vi "get_base_frequency.vi"(8 "error in (no error)":errorcluster, 11 "DL090211FPGAWrapper in":refnum<class "FPGAWrapperDL090211Galvo_grabber.lvclass">) -> (0 "error out":errorcluster, 2 "base frequency":dbl[unit]=40000000.0, 3 "DL090211FPGAWrapper out":refnum<class "FPGAWrapperDL090211Galvo_grabber.lvclass">)   [LabVIEW 2010, in "FPGAWrapperDL090211Galvo_grabber.lvclass"]
uses:
  FPGAWrapperDL090211Galvo_grabber.lvclass
  GenericFPGAWrapper/GenericFPGAWrapper/GenericFPGAWrapper.lvclass
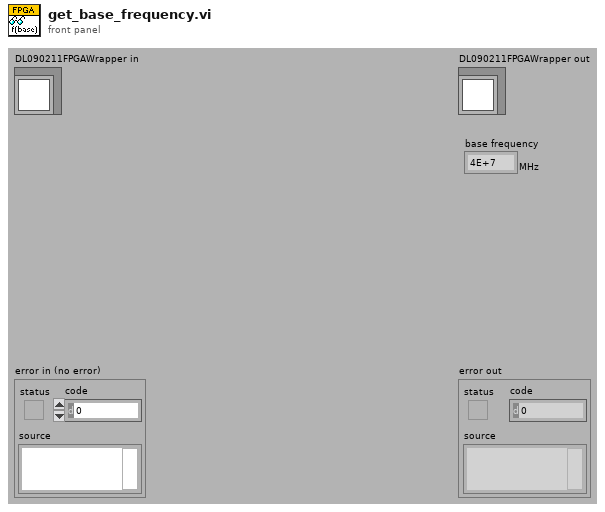
[diagram p1: front panel]
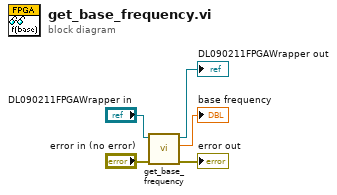
[diagram p0: block diagram]
diagram:
  n1 = call-parent "get_base_frequency.vi"("error in (no error)"="error in (no error)", "GenericFPGAWrapper in"="DL090211FPGAWrapper in") -> ("error out"=→"error out":errorcluster, "base frequency"=→"base frequency":dbl[unit], "GenericFPGAWrapper out"=→"DL090211FPGAWrapper out":refnum<class "FPGAWrapperDL090211Galvo_grabber.lvclass">)  [unwired: 7 in]
